vi "Lab1Code.vi"() -> ()   [LabVIEW 2015]
uses:
  <instrlib>/Stanford Research 830/Public/Data/Read (1 Parameter).vi
  <instrlib>/Stanford Research 830/Stanford Research 830.lvlib
panel:
  in  "Parameter (1: X)":u16(ring)=1 items=["X"=1, "Y"=2, "R"=3, "Theta"=4, "Channel 1"=5, "Channel 2"=6, "Aux In 1"=7, "Aux In 2"=8, "Aux In 3"=9, "Aux In 4"=10]
  out "Waveform Chart":dbl(graph)
  out "Amplitude/Phase Shift":dbl format="%#_3f"
  in  "Step Value":dbl=1000.0 min=1e-06 max=160000000.0 step=1.0 format="%#.6g"
  in  "Stop Value":dbl=1000.0 min=1e-06 max=160000000.0 step=1.0 format="%#.6g"
  in  "Start Value":dbl=1000.0 min=1e-06 max=160000000.0 step=1.0 format="%#.6g"
  in  "Reset (True)":bool=TRUE
  in  "error in (no error)":errorcluster
  in  "Lock in Amp":refnum<visa-resource-name>
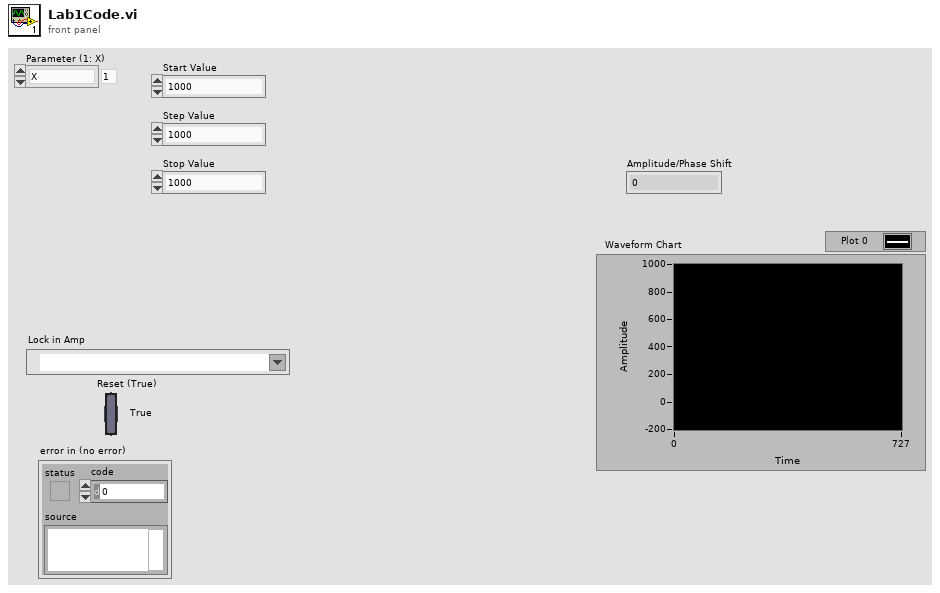
[diagram p1: front panel]
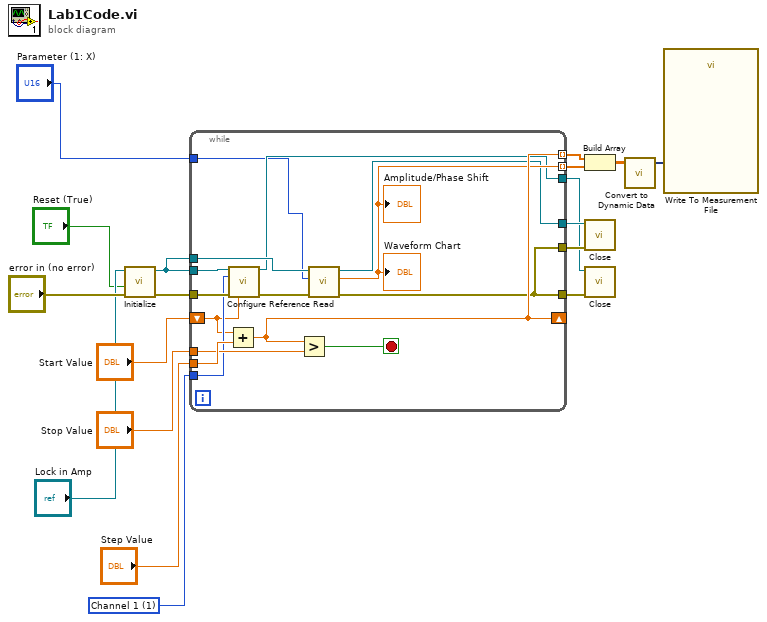
[diagram p0: block diagram]
diagram:
  w18 = 1 items=["Channel 1"=1, "Channel 2"=2] ("Channel (1:Channel 1)")
  n1 = call <instrlib>:"Initialize.vi"("error in (no error)"="error in (no error)", "Reset (True)"="Reset (True)", "VISA resource name"="Lock in Amp") -> ("error out"=w9:errorcluster, "VISA resource name out"=w2:refnum<visa-resource-name>)  [unwired: 7 in]
  n2 = while {
    tunnel: w18 -> [w25]
    tunnel: w9 -> [w28]
    tunnel: w2 -> [w26]
    tunnel: "Step Value" -> [w33]
    tunnel: "Stop Value" -> [w32]
    shift-right: [w31] -> _
    shift-left: "Start Value" -> [w24]
    tunnel: [w29] -> w14 mode=indexing
    tunnel: [w31] -> w13 mode=indexing
    tunnel: [w20] -> w8
    tunnel: w2 -> [w27]
    tunnel: [w22] -> w6
    tunnel: [w21] -> w5
    tunnel: "Parameter (1: X)" -> [w19]
    tunnel: [w20] -> w3
    stop <- w30 stop-if-true
    n3 = Add(x=w24, y=w33) -> (x+y=w31:dbl)
    n4 = call <instrlib>:"Configure Reference.vi"("VISA resource name"=w27, "Reference Source (1: Internal)"=w25, "error in (no error)"=w28, "Internal Reference Frequency (1000 Hz)"=w24) -> ("VISA resource name out"=w21:refnum<visa-resource-name>, "error out"=w23:errorcluster)  [unwired: 10 in]
    n5 = Greater?(x=w31, y=w32) -> (0:w30:bool)
    n6 = call-poly <instrlib>:"Read.vi"("error in (no error)"=w23, "Parameter (1: X)"=w19, "VISA resource name"=w26) -> ("error out"=w20:errorcluster, "Measurement"=w29:dbl, "VISA resource name out"=w22:refnum<visa-resource-name>)  [unwired: 6 in]
    "Amplitude/Phase Shift" <- w29
    "Waveform Chart" <- w29
  }
  n7 = Build Array(w13, w14) -> (w12:dbl[][])
  n8 = call <instrlib>:"Close.vi"("error in (no error)"=w8, "VISA resource name"=w6) -> ()  [unwired: 9 in, 1 out]
  n9 = call <instrlib>:"Close.vi"("error in (no error)"=w3, "VISA resource name"=w5) -> ()  [unwired: 9 in, 1 out]
  n10 = call "Convert to Dynamic Data"("2D Array"=w12) -> ("Dynamic Data Type"=w11:dynamicdata)  [unwired: 3 in]
  n11 = call "Write To Measurement File"("Signals"=w11) -> ()  [unwired: 16 in, 3 out]
